vi "Drive Direct.vi"(8 "error in":errorcluster, 9 "Left Wheel Velocity (mm/s)":i16, 10 "Right Wheel Velocity (mm/s)":i16, 11 "UART port in":T1) -> (0 "error out":errorcluster, 3 "UART port out":T1)   [LabVIEW 2014]
doc: "Directly actuate left and right wheels.\n\nThis VI writes to, but does not read from, the serial port."
uses:
  Advanced/UART/iRobot UART Port Type.ctl
  Advanced/Command/OpCode.ctl
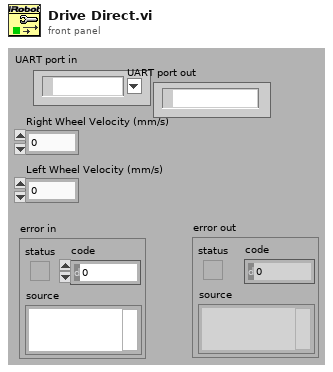
[diagram p1: front panel]
types:
  T1 = typedef "iRobot UART Port Type.ctl" = refnum<visa-resource-name>
  T2 = typedef "OpCode.ctl" = u8
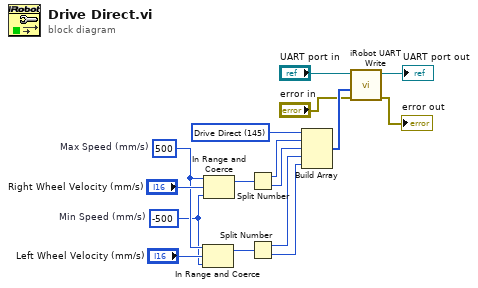
[diagram p0: block diagram]
diagram:
  w6 = i16 -500  # Min Speed (mm/s)
  w7 = i16 500  # Max Speed (mm/s)
  w9 = T2 145 items=["Start"=128, "Baud"=129, "Control"=130, "Safe"=131, "Full"=132, "Demo"=136, "Demo - Cover"=135, "Demo - Cover and Dock"=143, "Demo - Spot"=134, "Drive"=137, "Drive Direct"=145, "LEDs"=139, "Digital Outputs"=147, "PWM Low Side Drivers"=144, "Low Side Drivers"=138, "Send IR"=151, "Song"=140, "Play Song"=141, "Sensors"=142, "Query List"=149, "Stream"=148, "Pause/Resume Stream"=150, "Script"=152, "Play Script"=153, "Show Script"=154, "Wait Time"=155, "Wait Distance"=156, "Wait Angle"=157, "Wait Event"=158] ("OpCode")
  n1 = In Range and Coerce(upper limit=w7, x="Left Wheel Velocity (mm/s)", lower limit=w6) -> (coerced(x)=w8:i16)  [unwired: 1 out]
  n2 = In Range and Coerce(upper limit=w7, x="Right Wheel Velocity (mm/s)", lower limit=w6) -> (coerced(x)=w15:i16)  [unwired: 1 out]
  n3 = Split Number(x=w15) -> (hi(x)=w14:u8, lo(x)=w13:u8)
  n4 = Split Number(x=w8) -> (hi(x)=w11:u8, lo(x)=w10:u8)
  n5 = Build Array(w9, w14, w13, w11, w10) -> (w5:T2[])
  n6 = call "iRobot UART Write.vi"("error in"="error in", "data"=w5, "UART port in"="UART port in") -> ("error out"=→"error out":errorcluster, "UART port out"=→"UART port out":T1)  [unwired: 1 in, 6 out]
